vi "Write Report.vi"(8 "error in (no error)":errorcluster, 10 "Resource In":variant, 11 "Analyze Results Second Momentum in":refnum<class "Analyze Results Second Momentum.lvclass">) -> (0 "error out":errorcluster, 2 "Resource Out":variant, 3 "Analyze Results Second Momentum out":refnum<class "Analyze Results Second Momentum.lvclass">)   [LabVIEW 2014, in "Analyze Results Second Momentum.lvclass"]
uses:
  Analyze Results Second Momentum.lvclass
  <vilib>/Utility/config.llb/Config Data RefNum.ctl
  Results Base/Analyze Results Base.lvclass/Analyze Results Base.ctl
  Analyze Results Second Momentum.lvclass/Analyze Results Second Momentum.ctl
  Results Base/Read Section.vi
  Read 1st M x 1.vi
  Read 1st M y 1.vi
  Read 2nd M x 1.vi
  Read 2nd M y 1.vi
  Read D x 1.vi
  Read D y 1.vi
  <vilib>/Utility/config.llb/Write Key (Double).vi
  Results Base/Analyze Results Base.lvclass
  <vilib>/Utility/config.llb/NI_LVConfig.lvlib
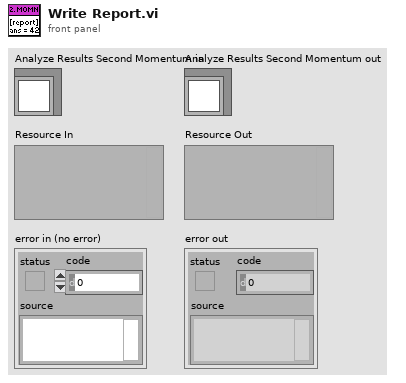
[diagram p1: front panel]
types:
  T1 = typedef "NI_LVConfig.lvlib/Config Data RefNum.ctl" = refnum<k1>
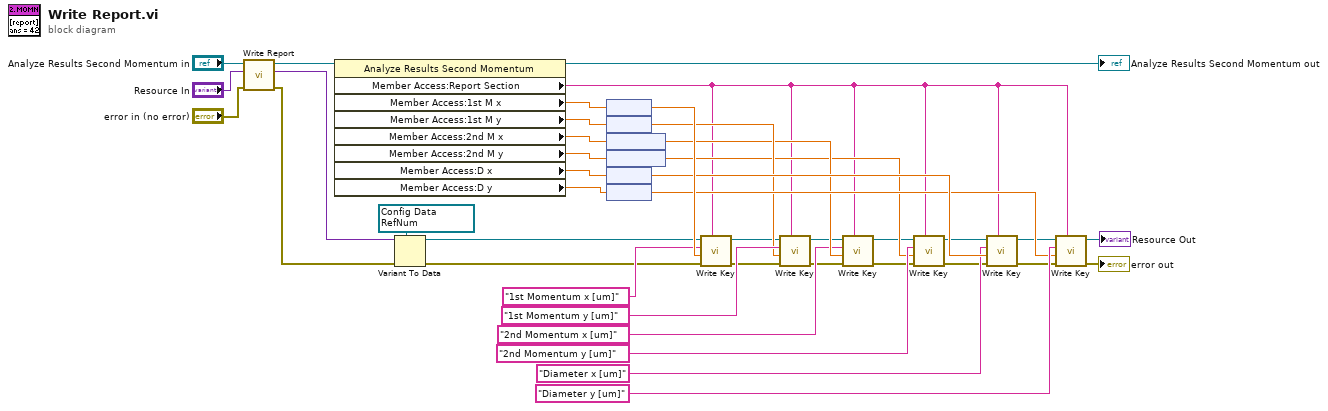
[diagram p0: block diagram]
diagram:
  w33 = T1 refnum items=["config data"] ("refnum")
  n1 = call-parent "Write Report.vi"("error in (no error)"="error in (no error)", "Resource In"="Resource In", "Analyze Results Base in"="Analyze Results Second Momentum in") -> ("error out"=w25:errorcluster, "Resource Out"=w34:variant, "Analyze Results Base out"=w38:refnum<class "Analyze Results Second Momentum.lvclass">)  [unwired: 6 in]
  n2 = property class="Analyze Results Second Momentum"(reference=w38) -> (reference out=→"Analyze Results Second Momentum out":refnum<class "Analyze Results Second Momentum.lvclass">, "Member Access:Report Section"=w8:string, "Member Access:1st M x"=w36:dbl[unit], "Member Access:1st M y"=w21:dbl[unit], "Member Access:2nd M x"=w19:dbl[unit], "Member Access:2nd M y"=w13:dbl[unit], "Member Access:D x"=w29:dbl[unit], "Member Access:D y"=w26:dbl[unit])  [unwired: 1 in, 1 out]
  n3 = Variant To Data(error in=w25, type=w33, Variant=w34) -> (data=w7:T1, error out=w24:errorcluster)
  n4 = node(w36) -> (w35:dbl)
  n5 = node(w21) -> (w22:dbl)
  n6 = node(w19) -> (w20:dbl)
  n7 = node(w13) -> (w14:dbl)
  n8 = node(w29) -> (w31:dbl)
  n9 = node(w26) -> (w27:dbl)
  n10 = call-poly <vilib>:"Write Key.vi"("section"=w8, "error in (no error)"=w24, "value"=w35, "key"="1st Momentum x [um]", "refnum"=w7) -> ("error out"=w17:errorcluster, "refnum out"=w6:T1)  [unwired: 4 in, 1 out]
  n11 = call-poly <vilib>:"Write Key.vi"("section"=w8, "error in (no error)"=w17, "value"=w22, "key"="1st Momentum y [um]", "refnum"=w6) -> ("error out"=w16:errorcluster, "refnum out"=w5:T1)  [unwired: 4 in, 1 out]
  n12 = call-poly <vilib>:"Write Key.vi"("section"=w8, "error in (no error)"=w16, "value"=w20, "key"="2nd Momentum x [um]", "refnum"=w5) -> ("error out"=w12:errorcluster, "refnum out"=w4:T1)  [unwired: 4 in, 1 out]
  n13 = call-poly <vilib>:"Write Key.vi"("section"=w8, "error in (no error)"=w12, "value"=w14, "key"="2nd Momentum y [um]", "refnum"=w4) -> ("error out"=w11:errorcluster, "refnum out"=w3:T1)  [unwired: 4 in, 1 out]
  n14 = call-poly <vilib>:"Write Key.vi"("section"=w8, "error in (no error)"=w11, "value"=w31, "key"="Diameter x [um]", "refnum"=w3) -> ("error out"=w10:errorcluster, "refnum out"=w2:T1)  [unwired: 4 in, 1 out]
  n15 = call-poly <vilib>:"Write Key.vi"("section"=w8, "error in (no error)"=w10, "value"=w27, "key"="Diameter y [um]", "refnum"=w2) -> ("error out"=→"error out":errorcluster, "refnum out"=→"Resource Out":T1)  [unwired: 4 in, 1 out]
